vi "modify 1 servo.vi"() -> ()   [LabVIEW 2012]
uses:
  <vilib>/Motion/FlexMotion/FunctionsVIs/AxisResourceConfig.llb/Enable Axes (8 axes).flx
  <vilib>/Motion/FlexMotion/FunctionsVIs/Trajectory.llb/Load Accel/Decel in RPS/sec.flx
  <vilib>/Motion/FlexMotion/FunctionsVIs/Trajectory.llb/Check Move Complete Status (8 axes).flx
  <vilib>/Motion/FlexMotion/FunctionsVIs/StartStopMotion.llb/Start Motion (8 axes).flx
  <vilib>/Motion/FlexMotion/FunctionsVIs/StartStopMotion.llb/Stop Motion (8 axes).flx
panel:
  in  "STOP":bool
  in  "VELOCITY in RPM":dbl=10.0
  in  "CHANGE DIRECTION":bool
  in  "RUN":bool
  in  "Value (200)":dbl=200.0 format="%.2f"
  in  "CHOOSE AXIS":T1={"AXIS1"=FALSE, "AXIS 2"=TRUE, "AXIS 3"=FALSE, "AXIS 4"=FALSE, "AXIS 5"=FALSE, "AXIS 6"=FALSE, "AXIS 7"=FALSE, "AXIS 8"=FALSE}
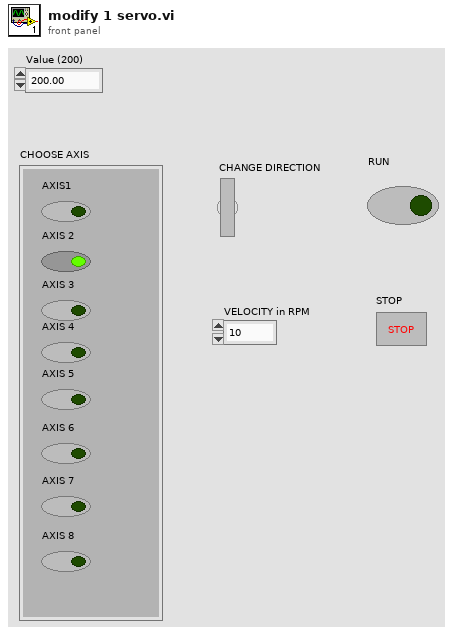
[diagram p1: front panel]
types:
  T1 = cluster{"AXIS1":bool, "AXIS 2":bool, "AXIS 3":bool, "AXIS 4":bool, "AXIS 5":bool, "AXIS 6":bool, "AXIS 7":bool, "AXIS 8":bool}
  T2 = enum16{"Absolute Position", "Relative Position", "Velocity", "Relative to Cap Pos", "Modulus Position", "Absolute Contouring", "Relative Contouring"}
  T3 = typedef "Board Id" = u8
  T4 = typedef "Bd Id Out" = u8
  T5 = typedef "Resource Out (Enum).flx" = u16
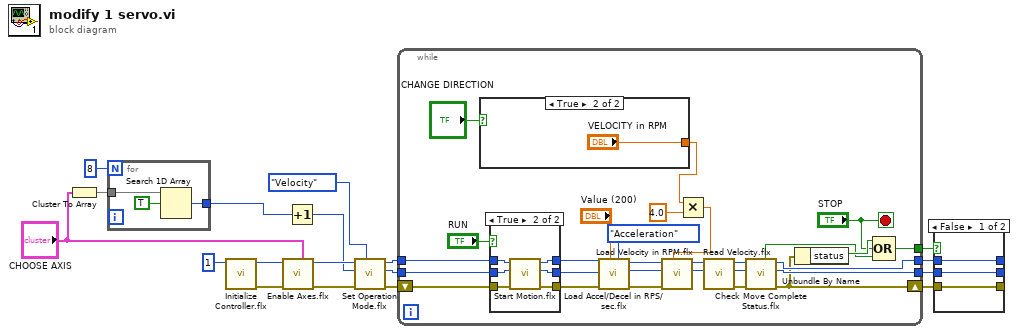
[diagram p0: block diagram]
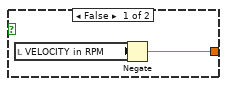
[diagram p3: hidden frame]
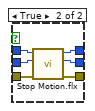
[diagram p4: hidden frame]
diagram:
  n1 = Cluster To Array(cluster="CHOOSE AXIS") -> (array=w4:bool[])
  n2 = for {
    N: 8 -> [_]
    tunnel: w4 -> [w21]
    tunnel: [w19] -> w3
    n3 = Search 1D Array(1D array=w21, element=TRUE) -> (index of element=w19:i32)  [unwired: 1 in]
  }
  n4 = call <vilib>:"Initialize Controller.flx"("Board ID"=T3 1) -> ("error out"=w16:errorcluster, "Bd ID Out"=w17:T4)  [unwired: 7 in]
  n5 = call-poly <vilib>:"Enable Axes.flx"("Axis Bitmap (Disabled)"="CHOOSE AXIS", "error in (no error)"=w16, "Board ID"=w17) -> ("error out"=w15:errorcluster, "Bd ID Out"=w14:T4)  [unwired: 5 in]
  n6 = Increment(x=w3) -> (x+1=w2:i32)
  n7 = call <vilib>:"Set Operation Mode.flx"("Position Mode (Absolute)"=T2."Velocity", "error in (no error)"=w15, "Axis or Vector Space"=w2, "Board ID"=w14) -> ("error out"=w10:errorcluster, "Resource Output"=w11:T5, "Bd ID Out"=w12:T4)  [unwired: 2 in]
  n8 = while {
    shift-right: [w39] -> w7
    shift-left: w10 -> [w35]
    tunnel: [w42] -> w6
    tunnel: w12 -> [w38]
    tunnel: w11 -> [w37]
    tunnel: [w41] -> w9
    tunnel: [w40] -> w8
    stop <- "STOP" stop-if-true
    n9 = case shown="True" "CHANGE DIRECTION" {
      tunnel: [w59 "VELOCITY in RPM"] -> w32
      frame False {
        n10 = local read "VELOCITY in RPM"() -> (w60:dbl)
        n11 = Negate(x=w60) -> (-x=w59:dbl)
      }
      frame True {
      }
    }
    n12 = case shown="True" "RUN" {
      tunnel: w38 -> [w52 w58]
      tunnel: w37 -> [w51 w57]
      tunnel: [w52 w56] -> w29
      tunnel: [w51 w55] -> w28
      tunnel: w35 -> [w50 w54]
      tunnel: [w50 w53] -> w27
      frame False {
      }
      frame True {
        n13 = call-poly <vilib>:"Start Motion.flx"("error in (no error)"=w54, "Axis or Vector Space"=w57, "Board ID"=w58) -> ("error out"=w53:errorcluster, "Resource Output"=w55:T5, "Bd ID Out"=w56:T4)  [unwired: 3 in]
      }
    }
    n14 = call "Load Accel/Decel in RPS/sec.flx"("Selector (Both)"=enum16{"Both", "Acceleration", "Deceleration"}."Acceleration", "Value (200)"="Value (200)", "error in (no error)"=w27, "Axis or Vector Space"=w28, "Board ID"=w29) -> ("error out"=w22:errorcluster, "Resource Output"=w23:T5, "Bd ID Out"=w24:T4)  [unwired: 2 in]
    n15 = Multiply(x=w32, y=4.0) -> (x*y=w31:dbl)
    n16 = call <vilib>:"Load Velocity in RPM.flx"("Velocity (500)"=w31, "error in (no error)"=w22, "Axis or Vector Space"=w23, "Board ID"=w24) -> ("Resource Output"=w43:T5, "Bd ID Out"=w44:T4)  [unwired: 3 in, 1 out]
    n17 = call <vilib>:"Read Velocity.flx"("Axis or Vector Space"=w43, "Board ID"=w44) -> ("error out"=w47:errorcluster, "Resource Output"=w48:T5, "Bd ID Out"=w49:T4)  [unwired: 4 in, 1 out]
    n18 = call-poly <vilib>:"Check Move Complete Status.flx"("error in (no error)"=w47, "Axis or Vector Space"=w48, "Board ID"=w49) -> ("error out"=w39:errorcluster, "Resource Output"=w40:T5, "Bd ID Out"=w41:T4, "Move Complete"=w45:bool)  [unwired: 3 in]
    n19 = Unbundle By Name(w39) -> ("status"=w46:bool)
    n20 = Compound Arithmetic op=OR(w46, "STOP", w45) -> (w42:bool)
  }
  n21 = case shown="False" w6 {
    tunnel: [w62 w70] -> _
    tunnel: [w64 w69] -> _
    tunnel: [w63 w68] -> _
    tunnel: w9 -> [w64 w67]
    tunnel: w8 -> [w63 w66]
    tunnel: w7 -> [w62 w65]
    frame False {
    }
    frame True {
      n22 = call-poly <vilib>:"Stop Motion.flx"("error in (no error)"=w65, "Axis or Vector Space"=w66, "Board ID"=w67) -> ("error out"=w70:errorcluster, "Resource Output"=w68:T5, "Bd ID Out"=w69:T4)  [unwired: 4 in]
    }
  }
